vi "Main_02A.vi"() -> ()   [LabVIEW 2025]
uses:
  <vilib>/Utility/error.llb/Trim Whitespace One-Sided.vi
  Utility/Universal Utility/TypeDefs_Utility/Cluster_Row-Column.ctl
  9e3f57c0-2ef8-4495-8287-c6a42a5fb955.vi
  Utility/Universal Utility/TypeDefs_Utility/ENUM_4 Directions U-D-L-R.ctl
  Utility/Universal Utility/TypeDefs_Utility/ENUM_8 Directions U-D-L-R.ctl
panel:
  out "U64 -1":u64
  out "Reject Array":u64[](array[numeric])
  out "MATCH":bool
  in  "Select Data":enum32{"Example", "Puzzle"}(tab)
  in  "EX Target":u64=1227775554
  in  "Example":string="11-22,95-115,998-1012,1188511880-1188511890,222220-222224,\n1698522-1698528,446443-446449,38593856-38593862,565653-565659,\n824824821-824824827,2121212118-2121212124"
  in  "Puzzle":string="874324-1096487,6106748-6273465,1751-4283,294380-348021,5217788-5252660,828815656-828846474,66486-157652,477-1035,20185-55252,17-47,375278481-375470130,141-453,33680490-33821359,88845663-88931344,621298-752726,21764551-21780350,58537958-58673847,9983248-10042949,4457-9048,9292891448-9292952618,4382577-4494092,199525-259728,9934981035-9935011120,6738255458-6738272752,8275916-8338174,1-15,68-128,7366340343-7366538971,82803431-82838224,72410788-72501583"
  in  "Puzzle Target":u64=43952536386
  out "Answer":u64
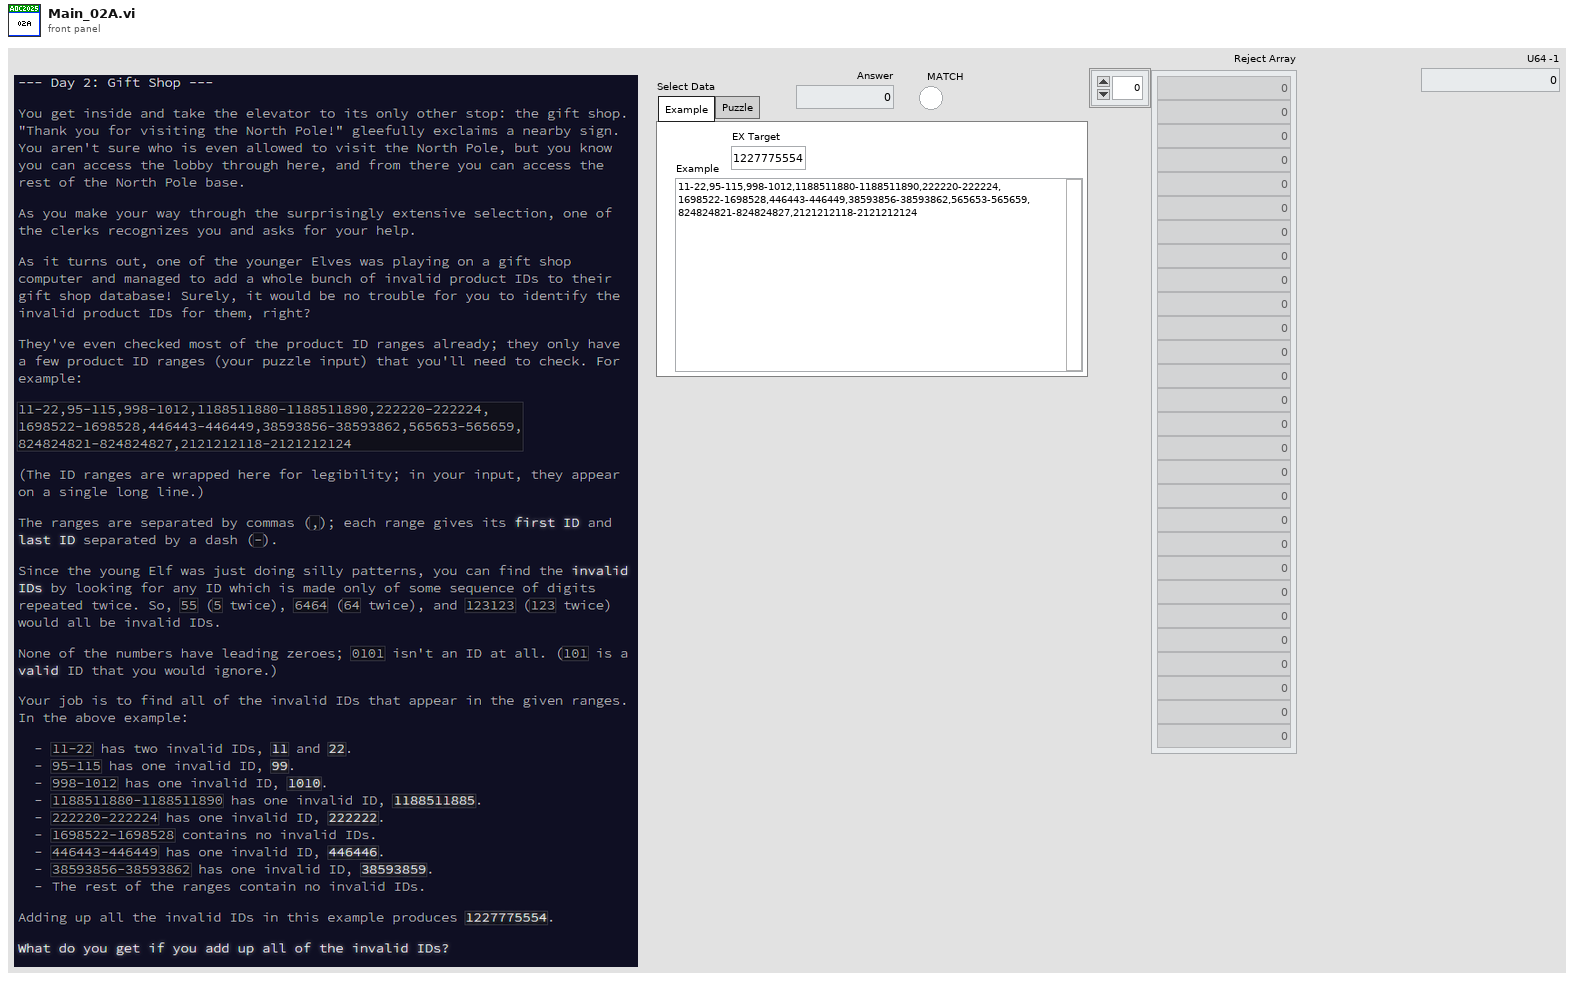
[diagram p1: front panel]
types:
  T1 = typedef "ENUM_8 Directions U-D-L-R.ctl" = enum16{"Up;-1,0", "Up-Right;-1,1", "Right;0,1", "Down-Right;1,1", "Down;1,0", "Down-Left;1,-1", "Left;0,-1", "Up-Left;-1,-1"}
  T2 = typedef "ENUM_4 Directions U-D-L-R.ctl" = enum16{"Up;-1,0", "Right;0,1", "Down;1,0", "Left;0,-1"}
  T3 = typedef "Cluster_Row-Column.ctl" = cluster{"R":i32, "C":i32}
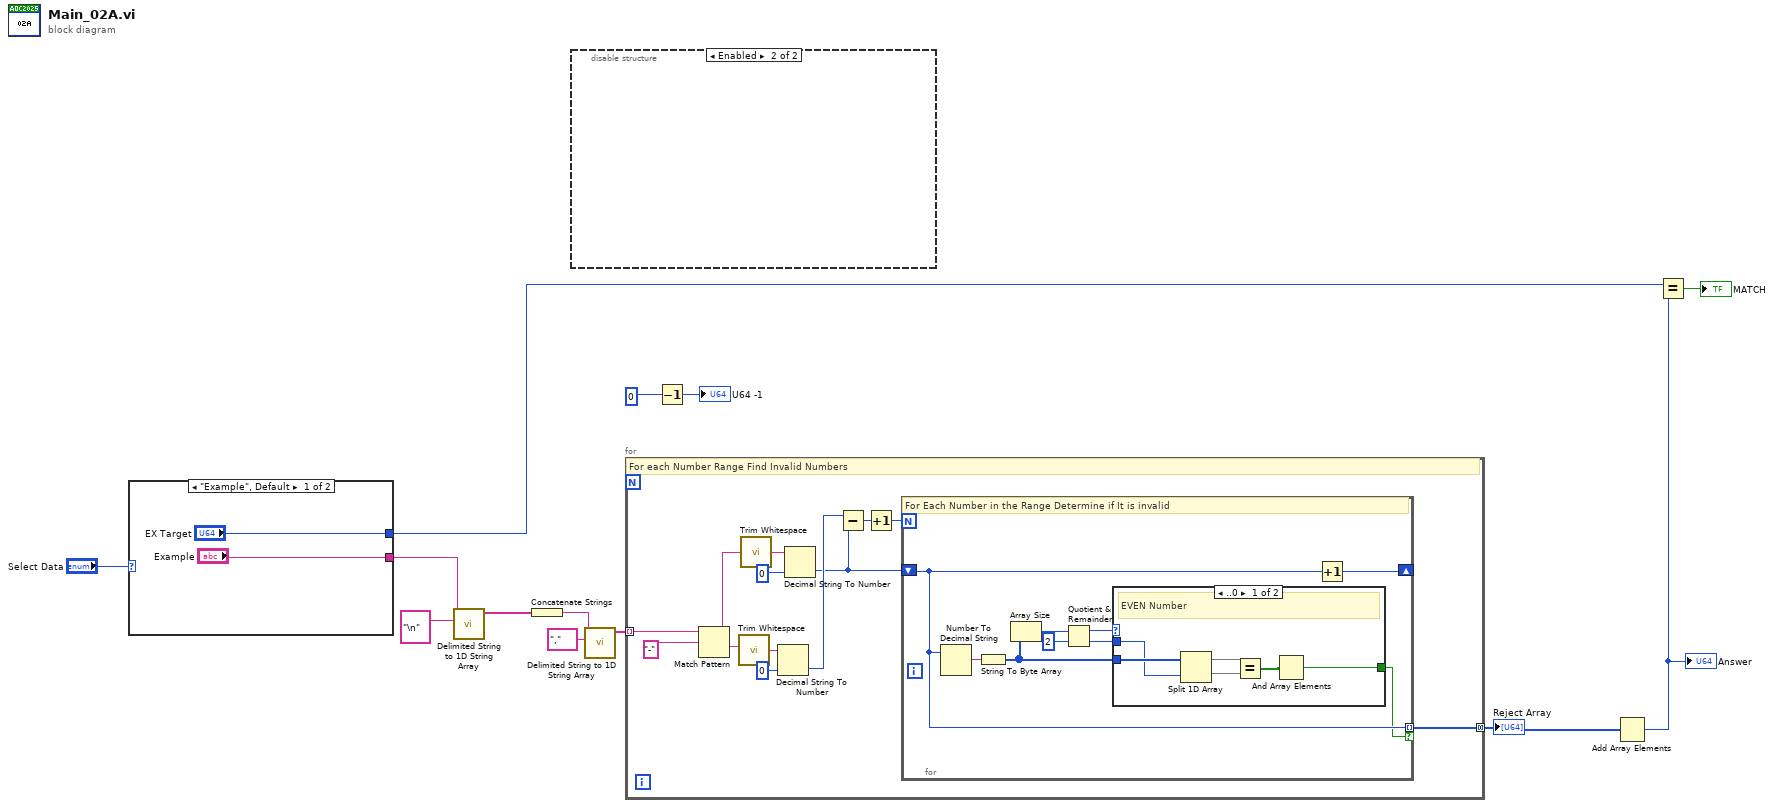
[diagram p0: block diagram]
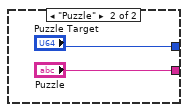
[diagram p2: hidden frame]
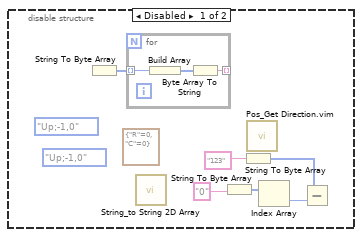
[diagram p3: hidden frame]
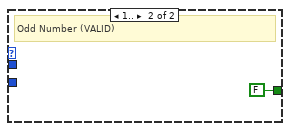
[diagram p4: hidden frame]
diagram:
  n1 = case shown="\"Example\", Default" "Select Data" {
    tunnel: ["Example" "Puzzle"] -> w2
    tunnel: ["EX Target" "Puzzle Target"] -> w9
    frame "Example", Default {
    }
    frame "Puzzle" {
    }
  }
  n2 = call <vilib>:"Delimited String to 1D String Array.vi"("delimiter"="\n" ("delimiter (Tab)"), "delimited string"=w2) -> ("string array"=w4:string[])  [unwired: 9 in]
  n3 = Concatenate Strings(w4) -> (w1:string)
  n4 = disable-structure shown="Enabled" {
    frame Disabled {
      (unwired) ENUM_8_Directions_U-D-L-R."Up;-1,0" ("Direction 8")
      (unwired) ENUM_4_Directions_U-D-L-R."Up;-1,0" ("Direction")
      (unwired) T3 {"R"=0, "C"=0} ("Position")
      n5 = String To Byte Array() -> (unsigned byte array=w18:u8[])  [unwired: 1 in]
      n6 = for {
        tunnel: w18 -> [w26] mode=indexing
        tunnel: [w24] -> _ mode=indexing
        n7 = Build Array(w26) -> (w25:u8[])
        n8 = Byte Array To String(unsigned byte array=w25) -> (string=w24:string)
      }
      n9 = call "String_to String 2D Array.vi"() -> ()  [unwired: 11 in, 1 out]
      n10 = String To Byte Array(string="0") -> (unsigned byte array=w21:u8[])
      n11 = String To Byte Array(string="123") -> (unsigned byte array=w19:u8[])
      n12 = call "Pos_Get Direction.vim"() -> ()  [unwired: 11 in, 1 out]
      n13 = Index Array(array=w21) -> (element=w20:u8)  [unwired: 1 in]
      n14 = Subtract(x=w19, y=w20) -> ()  [unwired: 1 out]
    }
    frame Enabled {
    }
  }
  n15 = call <vilib>:"Delimited String to 1D String Array.vi"("delimiter"="," ("delimiter (Tab)"), "delimited string"=w1) -> ("string array"=w12:string[])  [unwired: 9 in]
  n16 = for {
    tunnel: w12 -> [w39] mode=indexing
    tunnel: [w27] -> w8 mode=concatenating
    # "For each Number Range Find Invalid Numbers"
    n17 = Match Pattern(string=w39, regular expression="-" ("delimiter")) -> (before substring=w37:string, after substring=w35:string)  [unwired: 1 in, 2 out]
    n18 = call <vilib>:"Trim Whitespace.vi"("string"=w35) -> ("trimmed string"=w34:string)  [unwired: 1 in]
    n19 = call <vilib>:"Trim Whitespace.vi"("string"=w37) -> ("trimmed string"=w36:string)  [unwired: 1 in]
    n20 = Decimal String To Number(string=w34, default (0L)=u64 0 ("default (0 I32)")) -> (number=w31:u64)  [unwired: 1 in, 1 out]
    n21 = Decimal String To Number(string=w36, default (0L)=u64 0 ("default (0 I32)")) -> (number=w28:u64)  [unwired: 1 in, 1 out]
    n22 = Subtract(x=w31, y=w28) -> (x-y=w30:u64)
    n23 = Increment(x=w30) -> (x+1=w29:u64)
    n24 = for {
      N: w29 -> [_]
      shift-right: [w48] -> _
      shift-left: w28 -> [w44]
      tunnel: [w44] -> w27 mode=indexing if=w40
      # "For Each Number in the Range Determine if It is invalid"
      n25 = Number To Decimal String(number=w44) -> (decimal integer string=w43:string)  [unwired: 1 in]
      n26 = String To Byte Array(string=w43) -> (unsigned byte array=w41:u8[])
      n27 = Array Size(array=w41) -> (size(s)=w47:i32)
      n28 = Quotient & Remainder(x=w47, y=2) -> (x-y*floor(x/y)=w45:i32, floor(x/y)=w42:i32)
      n29 = case shown="..0" w45 {
        tunnel: w42 -> [w53 _]
        tunnel: w41 -> [w54 _]
        tunnel: [w49 FALSE] -> w40
        frame ..0 {
          # "EVEN Number"
          n30 = Split 1D Array(array=w54, index=w53) -> (first subarray=w52:u8[], second subarray=w51:u8[])
          n31 = Equal?(x=w52, y=w51) -> (x = y?=w50:bool[])
          n32 = And Array Elements(Boolean array=w50) -> (logical AND=w49:bool)
        }
        frame 1.. {
          # "Odd Number (VALID)"
        }
      }
      n33 = Increment(x=w44) -> (x+1=w48:u64)
    }
  }
  "Reject Array" <- w8
  n34 = Decrement(x=u64 0 ("sum")) -> (x-1=→"U64 -1":u64)
  n35 = Add Array Elements(numeric array=w8) -> (sum=w7:u64)
  "Answer" <- w7
  n36 = Equal?(x=w9, y=w7) -> (x = y?=→"MATCH":bool)
